vi "gen_carrier_channels.vi"(5 "Modulation info":T1 {"Hi channels at low" min=0 step=1; "Low carriers" format="%#_6p"; "High carriers" format="%#_6p"}, 7 "ilemt_config":T2 {"Filtering"."Distortion"."Limit" format="%#_3p"; "Filtering"."Distortion"."LF cut" format="%#_3p"; "Filtering"."Kalman"."Measure noise" format="%#_3p"; "Filtering"."Kalman"."Process noise" format="%#_3p"; "Filtering"."Hum"."Limit" format="%#_3p"; "Filtering"."Hum"."Frequency" format="%#_4p"; "Low rate STFT"."Oversample" min=1 step=1; "Low rate STFT"."Channels" min=0 step=1; "Low rate STFT"."DFT size" min=1 step=1; "Low rate STFT"."Window type" items=["Rectangle"=0, "Hanning"=1, "Hamming"=2, "Blackman-Harris"=3, "Exact Blackman"=4, "Blackman"=5, "Flat Top"=6, "4 Term B-Harris "=7, "7 Term B-Harris"=8, "Low Sidelobe"=9, "Blackman Nuttall"=11, "Triangle"=30, "Bartlett-Hanning"=31, "Bohman"=32, "Parzen"=33, "Welch"=34, "Kaiser"=60, "Dolph-Chebyshev"=61, "Gaussian"=62]; "High rate STFT"."Oversample" min=1 step=1; "High rate STFT"."Channels" min=0 step=1; "High rate STFT"."DFT size" min=1 step=1; "High rate STFT"."Window type" items=["Rectangle"=0, "Hanning"=1, "Hamming"=2, "Blackman-Harris"=3, "Exact Blackman"=4, "Blackman"=5, "Flat Top"=6, "4 Term B-Harris "=7, "7 Term B-Harris"=8, "Low Sidelobe"=9, "Blackman Nuttall"=11, "Triangle"=30, "Bartlett-Hanning"=31, "Bohman"=32, "Parzen"=33, "Welch"=34, "Kaiser"=60, "Dolph-Chebyshev"=61, "Gaussian"=62]; "IO params"."Carriers"."Levels" min=0.0 step=0.1; "IO params"."Conversion"."Rate" format="%#_8g"}, 10 "Source amplitudes":cdb[][][](array[numeric])) -> (3 "Carrier DFT":cdb[][](array[numeric]))   [LabVIEW 2014]
uses:
  ilemt_config.ctl
  system/IO_params.ctl
  stft_params.ctl
  <vilib>/Analysis/4window.llb/windowTd.ctl
  filter_params.ctl
  detrend_mode.ctl
  modulation_info.ctl
  <vilib>/Analysis/NI_AALPro.lvlib
panel:
  # "Generate carrier complex DFT using amplitudes specified by this array.  Page index is high/low carriers.  Row indicates the carrier frequency to generate (XYZ) and column is the source axis which the carrier is sent to.  This looks like the coupling matrix which is output from demodulation, but the interpretation is slightly different because we are concerned with off-axis signals in the source channels.   Our \"sensor\" is the current feedback, so the columns are tied to the source channels rather than the sensor.\n\nIdeally this array would be diagonal, with the X carrier only going to the X source axis, etc.  But cross-coupling happens due to output nonidealities. Specifying the desired carriers in this way allows us to generate (or cancel) off-axis carrier frequencies."
  # "X"
  # "Carriers"
  # "Y"
  # "Z"
  # "X"
  # "Y"
  # "Z"
  # "Source channels"
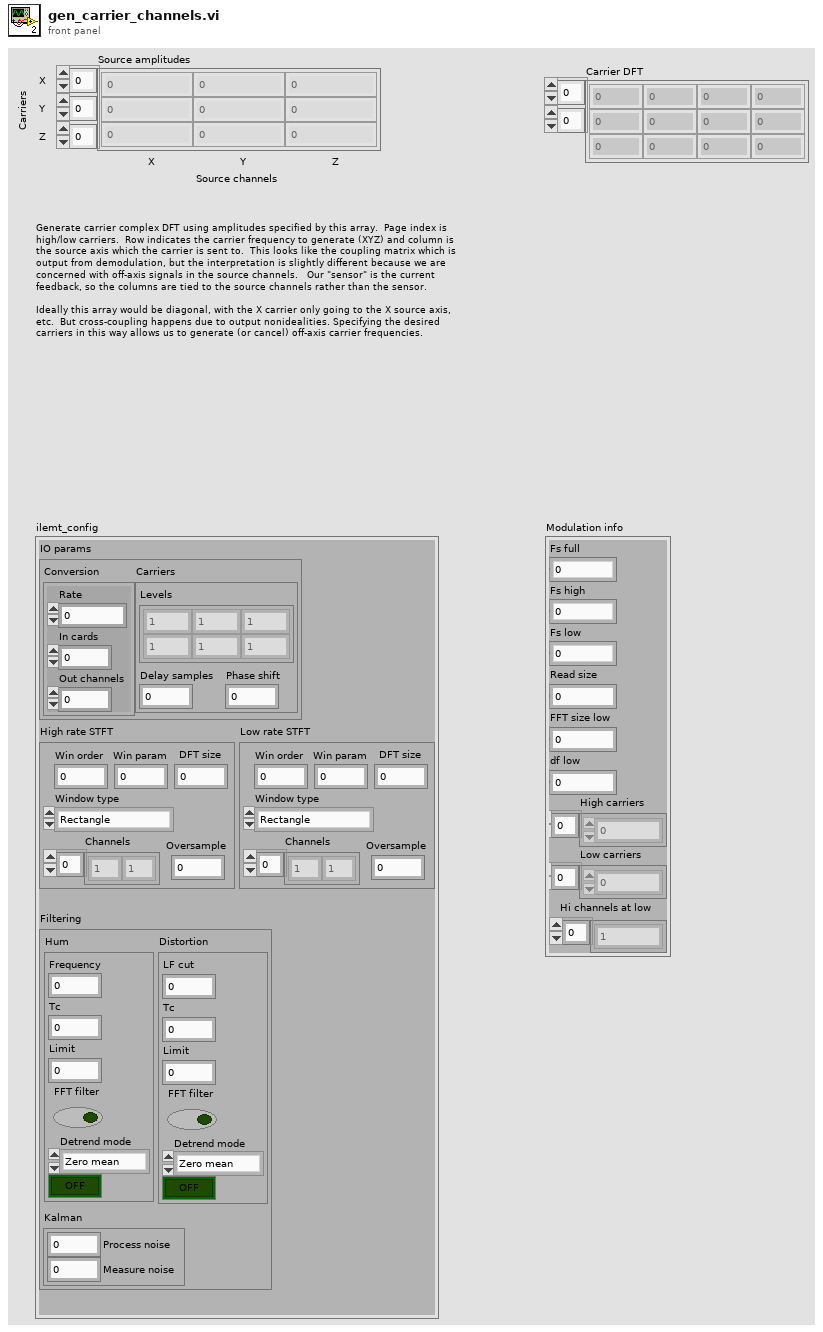
[diagram p1: front panel]
types:
  T1 = typedef "modulation_info.ctl" = cluster{"Fs full":dbl, "Fs high":dbl, "Fs low":dbl, "Read size":i32, "FFT size low":i32, "df low":dbl, "High carriers":dbl[], "Low carriers":dbl[], "Hi channels at low":i32[]}
  T2 = typedef "ilemt_config.ctl" = cluster{"IO params":T3, "High rate STFT":T4, "Low rate STFT":T4, "Filtering":T6}
  T3 = typedef "IO_params.ctl" = cluster{"Conversion":cluster{"Rate":dbl, "In cards":u32, "Out channels":u32}, "Carriers":cluster{"Phase shift":dbl, "Levels":dbl[][], "Delay samples":dbl}}
  T4 = typedef "stft_params.ctl" = cluster{"Win param":dbl, "Window type":T5, "Win order":i32, "DFT size":i32, "Channels":i32[], "Oversample":i32}
  T5 = typedef "NI_AALPro.lvlib/windowTd.ctl" = u32
  T6 = typedef "filter_params.ctl" = cluster{"Hum":cluster{"Frequency":dbl, "Tc":dbl, "Limit":dbl, "FFT filter":bool, "Detrend mode":T7, "Enable":bool}, "Kalman":cluster{"Process noise":dbl, "Measure noise":dbl}, "Distortion":cluster{"LF cut":dbl, "Tc":dbl, "Limit":dbl, "FFT filter":bool, "Detrend mode":T7, "Enable":bool}}
  T7 = typedef "detrend_mode.ctl" = enum16{"Zero mean", "Linear", "Robust linear"}
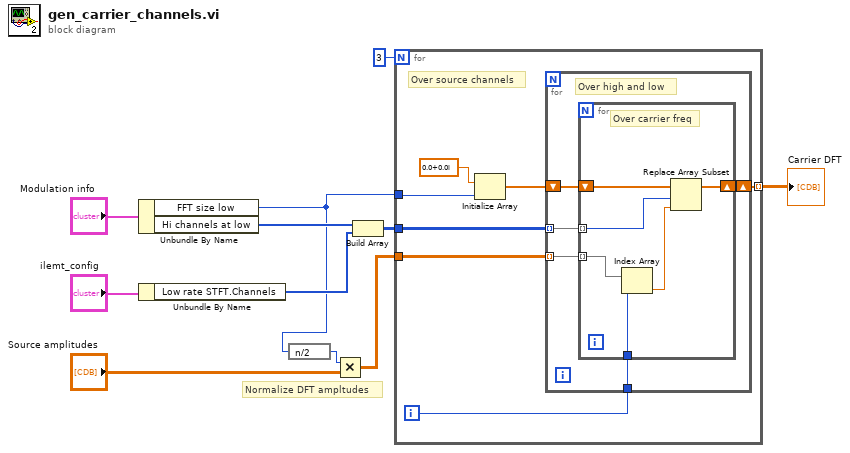
[diagram p0: block diagram]
diagram:
  # "Normalize DFT ampltudes"
  n1 = Unbundle By Name("Modulation info") -> ("FFT size low"=w1:i32, "Hi channels at low"=w6:i32[])
  n2 = Unbundle By Name("ilemt_config") -> ("Low rate STFT.Channels"=w5:i32[])
  n3 = expression code="n/2"(w1) -> (w9:i32)
  n4 = Multiply(x=w9, y="Source amplitudes") -> (x*y=w7:cdb[][][])
  n5 = Build Array(w6, w5) -> (w4:i32[][])
  n6 = for {
    N: 3 -> [_]
    tunnel: w1 -> [w16]
    tunnel: w7 -> [w15]
    tunnel: w4 -> [w14]
    tunnel: [w13] -> w3 mode=indexing
    i -> [w12]
    # "Over source channels"
    n7 = Initialize Array(cdb 0.0+0.0i, w16) -> (w17:cdb[])
    n8 = for {
      tunnel: w15 -> [w21] mode=indexing
      tunnel: w14 -> [w22] mode=indexing
      shift-right: [w20] -> w13
      shift-left: w17 -> [w23]
      tunnel: w12 -> [w19]
      # "Over high and low"
      n9 = for {
        tunnel: w22 -> [w28] mode=indexing
        tunnel: w21 -> [w26] mode=indexing
        shift-right: [w27] -> w20
        shift-left: w23 -> [w29]
        tunnel: w19 -> [w24]
        # "Over carrier freq"
        n10 = Index Array(array=w26, index=w24) -> (element=w25:cdb)
        n11 = Replace Array Subset(array=w29, new element=w25, index=w28) -> (w27:cdb[])
      }
    }
  }
  "Carrier DFT" <- w3
